vi "MSFET208_Temp_CalibCalc.vi"(11 "Voltage from Thermistor":dbl=0.8611887382361767) -> (2 "Temperature (C)":dbl=24.4655047055293)   [LabVIEW 2018]
panel:
  in  "calVoltage":dbl=0.8612
  in  "calTemp":dbl=22.71
  # "INPUTS"
  # "OUTPUTS"
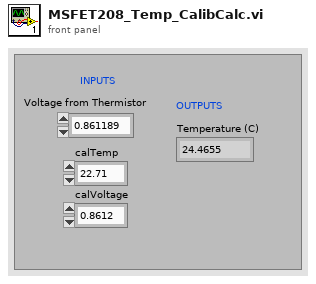
[diagram p1: front panel]
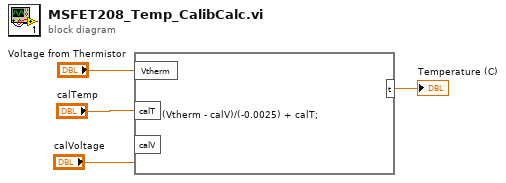
[diagram p0: block diagram]
diagram:
  n1 = formula code="t = (Vtherm - calV)/(-0.0025) + calT;"("Vtherm"="Voltage from Thermistor", "calT"="calTemp", "calV"="calVoltage") -> ("t"=→"Temperature (C)":dbl)
